vi "Load Enabled Settings.vi"(8 "Error in":errorcluster caption="Error in (no error)", 11 "Settings Path":path) -> (0 "Error out":errorcluster, 1 "Loaded Default?":bool, 3 "Enabled Sections":T1={"Projects"=TRUE, "Interfaces"=TRUE, "Classes"=TRUE, "Libraries"=TRUE, "VIs"=TRUE, "Controls"=TRUE, "LLBs"=TRUE})   [LabVIEW 2023, in "VIDoc Printer.lvlib" / "Printer Settings.lvclass"]
uses:
  Printer Settings.lvclass
  Enabled Sections Cluster.ctl
  ac5b38ed-98c3-46aa-8a0e-3b9f0d21d897.vi
  <vilib>/JDP Science/JSONtext/JSON text to Variant.vi
  <vilib>/JDP Science/JSONtext/LVClass Serializer/JSONtext LVClass Serializer.lvclass
  Printer Settings.lvclass/Printer Settings.ctl
  VIDoc Settings/VIDoc Settings.lvclass
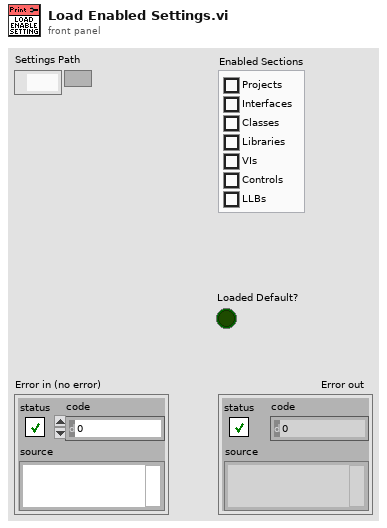
[diagram p1: front panel]
types:
  T1 = typedef "VIDoc Printer.lvlib/Printer Settings.lvclass/Enabled Sections Cluster.ctl" = cluster{"Projects":bool, "Interfaces":bool, "Classes":bool, "Libraries":bool, "VIs":bool, "Controls":bool, "LLBs":bool}
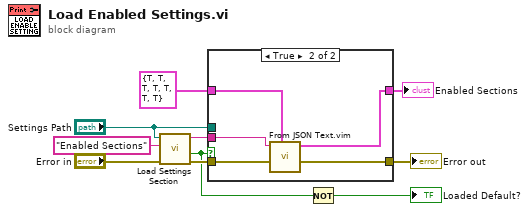
[diagram p0: block diagram]
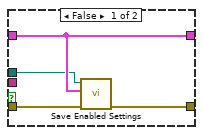
[diagram p2: hidden frame]
diagram:
  n1 = call "Load Settings Section.vi"("Error in"="Error in", "Section Name"="Enabled Sections", "JSON Settings Path"="Settings Path") -> ("Error out"=w8:errorcluster, "Found"=w3:bool, "JSON Object"=w7:string)  [unwired: 6 in]
  n2 = case shown="True" w3 {
    tunnel: w8 -> [w14 w19]
    tunnel: w7 -> [_ w18]
    tunnel: T1 {"Projects"=TRUE, "Interfaces"=TRUE, "Classes"=TRUE, "Libraries"=TRUE, "VIs"=TRUE, "Controls"=TRUE, "LLBs"=TRUE} ("Enabled Sections") -> [w12 w17]
    tunnel: [w12 w16] -> w1
    tunnel: [w13 w15] -> w5
    tunnel: "Settings Path" -> [w11 _]
    frame False {
      n3 = call "Save Enabled Settings.vi"("Error in"=w14, "Enabled Sections"=w12, "Settings Path"=w11) -> ("Error out"=w13:errorcluster)  [unwired: 8 in]
    }
    frame True {
      n4 = call "From JSON Text.vim"("Data Type and Default Value"=w17, "error in (no error)"=w19, "JSON"=w18) -> ("error out"=w15:errorcluster, "Data out"=w16:T1)  [unwired: 7 in]
    }
  }
  "Error out" <- w5
  "Enabled Sections" <- w1
  n5 = Not(x=w3) -> (.not. x?=→"Loaded Default?":bool)
